vi "ejemplo.vi"(9 "Numeric 3":dbl, 10 "Numeric 4":dbl, 11 "Numeric 5":dbl) -> (2 "Numeric":u8, 3 "Numeric 2":dbl)   [LabVIEW 2014]
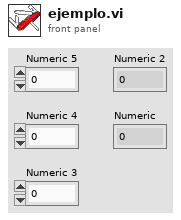
[diagram p1: front panel]
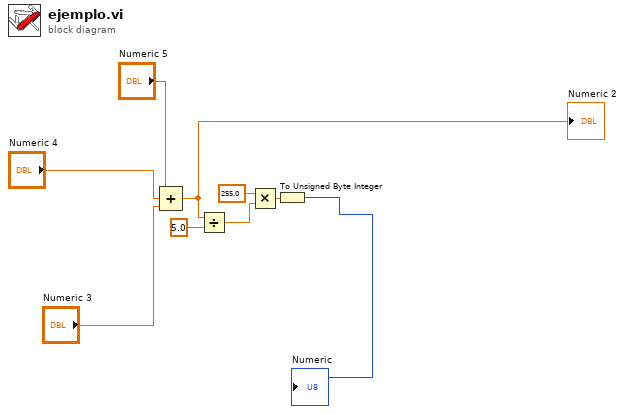
[diagram p0: block diagram]
diagram:
  n1 = Compound Arithmetic op=ADD("Numeric 5", "Numeric 4", "Numeric 3") -> (w8:dbl)
  "Numeric 2" <- w8
  n2 = Divide(x=w8, y=5.0) -> (x/y=w5:dbl)
  n3 = Multiply(x=255.0, y=w5) -> (x*y=w7:dbl)
  n4 = To Unsigned Byte Integer(number=w7) -> (unsigned 8bit integer=→"Numeric":u8)
